vi "VI Tree.vi"   [LabVIEW 2020, in "IT-M7700.lvlib"]
doc: "This is the instrument driver for the <INSTRUMENT NAME>. The VI Tree displays all the user-callable VIs of the instrument driver in an organized table."
uses:
  <instrlib>/IT-M7700/IT-M7700.lvlib
panel:
  # "(c) 2014 <Enter Company Name Here>.  ALL RIGHTS RESERVED."
  # "SEE DIAGRAM\nFOR VI TREE."
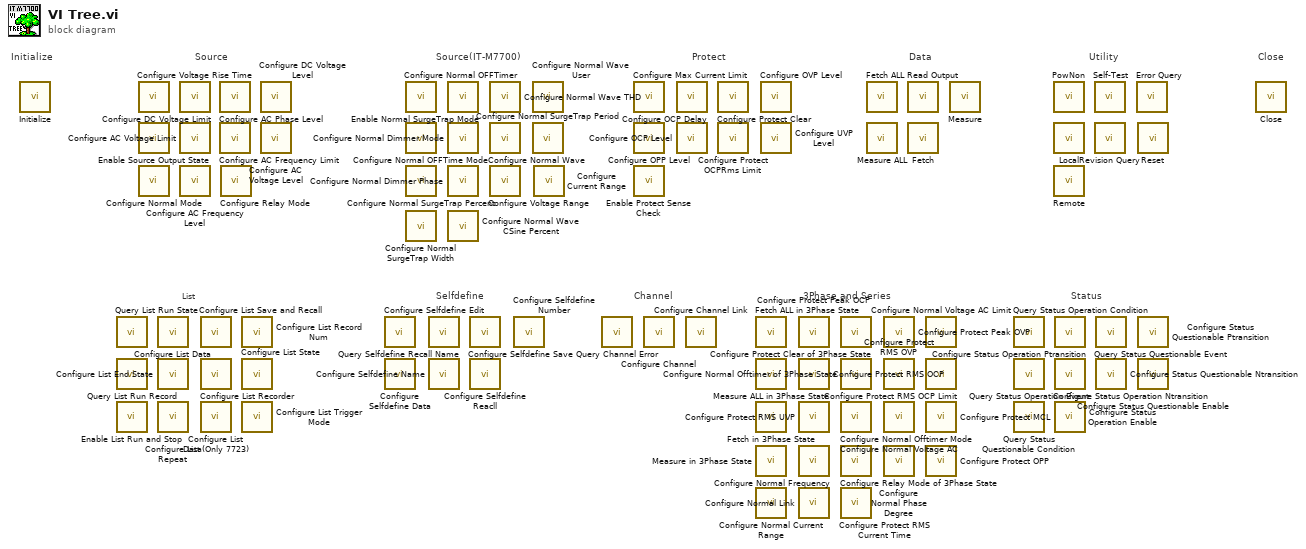
[diagram p0: block diagram]
diagram:
  # "Status"
  # "3Phase and Series"
  # "Channel"
  # "Selfdefine"
  # "Source(IT-M7700)"
  # "Protect"
  # "List"
  # "Source"
  # "Utility"
  # "Data"
  # "Close"
  # "Initialize"
  n1 = call <instrlib>:"Initialize.vi"() -> ()  [unwired: 10 in, 2 out]
  n2 = call <instrlib>:"Query List Run State.vi"() -> ()  [unwired: 9 in, 3 out]
  n3 = call <instrlib>:"Query List Run Record.vi"() -> ()  [unwired: 9 in, 3 out]
  n4 = call <instrlib>:"Enable List Run and Stop.vi"() -> ()  [unwired: 10 in, 2 out]
  n5 = call <instrlib>:"Configure Voltage Rise Time.vi"() -> ()  [unwired: 10 in, 2 out]
  n6 = call <instrlib>:"Enable Source Output State.vi"() -> ()  [unwired: 10 in, 2 out]
  n7 = call <instrlib>:"Configure Normal Mode.vi"() -> ()  [unwired: 10 in, 2 out]
  n8 = call <instrlib>:"Configure List Data.vi"() -> ()  [unwired: 10 in, 2 out]
  n9 = call <instrlib>:"Configure List End State.vi"() -> ()  [unwired: 10 in, 2 out]
  n10 = call <instrlib>:"Configure List Repeat.vi"() -> ()  [unwired: 10 in, 2 out]
  n11 = call <instrlib>:"Configure DC Voltage Limit.vi"() -> ()  [unwired: 10 in, 2 out]
  n12 = call <instrlib>:"Configure AC Voltage Limit.vi"() -> ()  [unwired: 10 in, 2 out]
  n13 = call <instrlib>:"Configure AC Frequency Level.vi"() -> ()  [unwired: 10 in, 2 out]
  n14 = call <instrlib>:"Configure List Save and Recall.vi"() -> ()  [unwired: 10 in, 2 out]
  n15 = call <instrlib>:"Configure List Recorder.vi"() -> ()  [unwired: 10 in, 2 out]
  n16 = call <instrlib>:"Configure List Data(Only 7723).vi"() -> ()  [unwired: 10 in, 2 out]
  n17 = call <instrlib>:"Configure AC Phase Level.vi"() -> ()  [unwired: 10 in, 2 out]
  n18 = call <instrlib>:"Configure AC Frequency Limit.vi"() -> ()  [unwired: 10 in, 2 out]
  n19 = call <instrlib>:"Configure Relay Mode.vi"() -> ()  [unwired: 10 in, 2 out]
  n20 = call <instrlib>:"Configure List Record Num.vi"() -> ()  [unwired: 10 in, 2 out]
  n21 = call <instrlib>:"Configure List State.vi"() -> ()  [unwired: 10 in, 2 out]
  n22 = call <instrlib>:"Configure List Trigger Mode.vi"() -> ()  [unwired: 10 in, 2 out]
  n23 = call <instrlib>:"Configure DC Voltage Level.vi"() -> ()  [unwired: 10 in, 2 out]
  n24 = call <instrlib>:"Configure AC Voltage Level.vi"() -> ()  [unwired: 10 in, 2 out]
  n25 = call <instrlib>:"Configure Selfdefine Edit.vi"() -> ()  [unwired: 10 in, 2 out]
  n26 = call <instrlib>:"Configure Selfdefine Data.vi"() -> ()  [unwired: 10 in, 2 out]
  n27 = call <instrlib>:"Configure Normal OFFTimer.vi"() -> ()  [unwired: 10 in, 2 out]
  n28 = call <instrlib>:"Configure Normal OFFTime Mode.vi"() -> ()  [unwired: 10 in, 2 out]
  n29 = call <instrlib>:"Configure Normal SurgeTrap Percent.vi"() -> ()  [unwired: 10 in, 2 out]
  n30 = call <instrlib>:"Configure Normal SurgeTrap Width.vi"() -> ()  [unwired: 10 in, 2 out]
  n31 = call <instrlib>:"Query Selfdefine Recall Name.vi"() -> ()  [unwired: 9 in, 3 out]
  n32 = call <instrlib>:"Configure Selfdefine Name.vi"() -> ()  [unwired: 10 in, 2 out]
  n33 = call <instrlib>:"Enable Normal SurgeTrap Mode.vi"() -> ()  [unwired: 10 in, 2 out]
  n34 = call <instrlib>:"Configure Normal Dimmer Mode.vi"() -> ()  [unwired: 10 in, 2 out]
  n35 = call <instrlib>:"Configure Normal Dimmer Phase.vi"() -> ()  [unwired: 10 in, 2 out]
  n36 = call <instrlib>:"Configure Normal Wave CSine Percent.vi"() -> ()  [unwired: 10 in, 2 out]
  n37 = call <instrlib>:"Configure Selfdefine Save.vi"() -> ()  [unwired: 10 in, 2 out]
  n38 = call <instrlib>:"Configure Selfdefine Reacll.vi"() -> ()  [unwired: 10 in, 2 out]
  n39 = call <instrlib>:"Configure Normal Wave THD.vi"() -> ()  [unwired: 10 in, 2 out]
  n40 = call <instrlib>:"Configure Normal Wave.vi"() -> ()  [unwired: 10 in, 2 out]
  n41 = call <instrlib>:"Configure Voltage Range.vi"() -> ()  [unwired: 10 in, 2 out]
  n42 = call <instrlib>:"Configure Selfdefine Number.vi"() -> ()  [unwired: 10 in, 2 out]
  n43 = call <instrlib>:"Configure Normal Wave User.vi"() -> ()  [unwired: 10 in, 2 out]
  n44 = call <instrlib>:"Configure Normal SurgeTrap Period.vi"() -> ()  [unwired: 10 in, 2 out]
  n45 = call <instrlib>:"Configure Current Range.vi"() -> ()  [unwired: 10 in, 2 out]
  n46 = call <instrlib>:"Query Channel Error.vi"() -> ()  [unwired: 9 in, 3 out]
  n47 = call <instrlib>:"Configure Max Current Limit.vi"() -> ()  [unwired: 10 in, 2 out]
  n48 = call <instrlib>:"Configure OPP Level.vi"() -> ()  [unwired: 10 in, 2 out]
  n49 = call <instrlib>:"Enable Protect Sense Check.vi"() -> ()  [unwired: 10 in, 2 out]
  n50 = call <instrlib>:"Configure Channel.vi"() -> ()  [unwired: 10 in, 2 out]
  n51 = call <instrlib>:"Configure OCP Delay.vi"() -> ()  [unwired: 10 in, 2 out]
  n52 = call <instrlib>:"Configure OCP Level.vi"() -> ()  [unwired: 10 in, 2 out]
  n53 = call <instrlib>:"Configure Channel Link.vi"() -> ()  [unwired: 10 in, 2 out]
  n54 = call <instrlib>:"Configure Protect Clear.vi"() -> ()  [unwired: 10 in, 2 out]
  n55 = call <instrlib>:"Configure Protect OCPRms Limit.vi"() -> ()  [unwired: 10 in, 2 out]
  n56 = call <instrlib>:"Fetch ALL in 3Phase State.vi"() -> ()  [unwired: 9 in, 3 out]
  n57 = call <instrlib>:"Measure ALL in 3Phase State.vi"() -> ()  [unwired: 9 in, 3 out]
  n58 = call <instrlib>:"Fetch in 3Phase State.vi"() -> ()  [unwired: 9 in, 3 out]
  n59 = call <instrlib>:"Measure in 3Phase State.vi"() -> ()  [unwired: 9 in, 3 out]
  n60 = call <instrlib>:"Configure Normal Current Range.vi"() -> ()  [unwired: 10 in, 2 out]
  n61 = call <instrlib>:"Configure OVP Level.vi"() -> ()  [unwired: 10 in, 2 out]
  n62 = call <instrlib>:"Configure UVP Level.vi"() -> ()  [unwired: 10 in, 2 out]
  n63 = call <instrlib>:"Configure Protect Peak OCP.vi"() -> ()  [unwired: 10 in, 2 out]
  n64 = call <instrlib>:"Configure Protect RMS OCP.vi"() -> ()  [unwired: 10 in, 2 out]
  n65 = call <instrlib>:"Configure Protect RMS UVP.vi"() -> ()  [unwired: 10 in, 2 out]
  n66 = call <instrlib>:"Configure Normal Frequency.vi"() -> ()  [unwired: 10 in, 2 out]
  n67 = call <instrlib>:"Configure Normal Link.vi"() -> ()  [unwired: 10 in, 2 out]
  n68 = call <instrlib>:"Configure Protect Clear of 3Phase State.vi"() -> ()  [unwired: 10 in, 2 out]
  n69 = call <instrlib>:"Configure Normal Offtimer of 3Phase State.vi"() -> ()  [unwired: 10 in, 2 out]
  n70 = call <instrlib>:"Configure Normal Offtimer Mode.vi"() -> ()  [unwired: 10 in, 2 out]
  n71 = call <instrlib>:"Configure Relay Mode of 3Phase State.vi"() -> ()  [unwired: 10 in, 2 out]
  n72 = call <instrlib>:"Configure Protect RMS Current Time.vi"() -> ()  [unwired: 10 in, 2 out]
  n73 = call <instrlib>:"Fetch ALL.vi"() -> ()  [unwired: 9 in, 3 out]
  n74 = call <instrlib>:"Measure ALL.vi"() -> ()  [unwired: 9 in, 3 out]
  n75 = call <instrlib>:"Configure Protect Peak OVP.vi"() -> ()  [unwired: 10 in, 2 out]
  n76 = call <instrlib>:"Configure Protect RMS OVP.vi"() -> ()  [unwired: 10 in, 2 out]
  n77 = call <instrlib>:"Configure Normal Voltage AC.vi"() -> ()  [unwired: 10 in, 2 out]
  n78 = call <instrlib>:"Configure Normal Phase Degree.vi"() -> ()  [unwired: 10 in, 2 out]
  n79 = call <instrlib>:"Read Output.vi"() -> ()  [unwired: 8 in, 4 out]
  n80 = call <instrlib>:"Fetch.vi"() -> ()  [unwired: 9 in, 3 out]
  n81 = call <instrlib>:"Configure Normal Voltage AC Limit.vi"() -> ()  [unwired: 10 in, 2 out]
  n82 = call <instrlib>:"Configure Protect RMS OCP Limit.vi"() -> ()  [unwired: 10 in, 2 out]
  n83 = call <instrlib>:"Configure Protect MCL.vi"() -> ()  [unwired: 10 in, 2 out]
  n84 = call <instrlib>:"Configure Protect OPP.vi"() -> ()  [unwired: 10 in, 2 out]
  n85 = call <instrlib>:"Measure.vi"() -> ()  [unwired: 9 in, 3 out]
  n86 = call <instrlib>:"Query Status Operation Condition.vi"() -> ()  [unwired: 9 in, 3 out]
  n87 = call <instrlib>:"Query Status Operation Event.vi"() -> ()  [unwired: 9 in, 3 out]
  n88 = call <instrlib>:"Query Status Questionable Condition.vi"() -> ()  [unwired: 9 in, 3 out]
  n89 = call <instrlib>:"PowNon.vi"() -> ()  [unwired: 10 in, 2 out]
  n90 = call <instrlib>:"Local.vi"() -> ()  [unwired: 10 in, 2 out]
  n91 = call <instrlib>:"Remote.vi"() -> ()  [unwired: 10 in, 2 out]
  n92 = call <instrlib>:"Configure Status Operation Ptransition.vi"() -> ()  [unwired: 10 in, 2 out]
  n93 = call <instrlib>:"Configure Status Operation Ntransition.vi"() -> ()  [unwired: 10 in, 2 out]
  n94 = call <instrlib>:"Configure Status Operation Enable.vi"() -> ()  [unwired: 10 in, 2 out]
  n95 = call <instrlib>:"Self-Test.vi"() -> ()  [unwired: 8 in, 4 out]
  n96 = call <instrlib>:"Revision Query.vi"() -> ()  [unwired: 8 in, 4 out]
  n97 = call <instrlib>:"Query Status Questionable Event.vi"() -> ()  [unwired: 9 in, 3 out]
  n98 = call <instrlib>:"Configure Status Questionable Ntransition.vi"() -> ()  [unwired: 10 in, 2 out]
  n99 = call <instrlib>:"Error Query.vi"() -> ()  [unwired: 8 in, 4 out]
  n100 = call <instrlib>:"Reset.vi"() -> ()  [unwired: 10 in, 2 out]
  n101 = call <instrlib>:"Configure Status Questionable Ptransition.vi"() -> ()  [unwired: 10 in, 2 out]
  n102 = call <instrlib>:"Configure Status Questionable Enable.vi"() -> ()  [unwired: 10 in, 2 out]
  n103 = call <instrlib>:"Close.vi"() -> ()  [unwired: 11 in, 1 out]
